vi "LoadStaticConfig.vi"(7 "UIMsg":refnum<class "SendMessage.lvclass">, 8 "error in (no error)":errorcluster, 11 "VXMMotionManager in":refnum<class "VXMMotionManager.lvclass">) -> (0 "error out":errorcluster, 3 "VXMMotionManager out":refnum<class "VXMMotionManager.lvclass">)   [LabVIEW 2018, in "VXMMotionManager.lvclass"]
uses:
  VXMMotionManager.lvclass
  SendMessage/SendMessage.lvclass
  MotionTypes.ctl
  VXMMotionManager.lvclass/VXMMotionManager.ctl
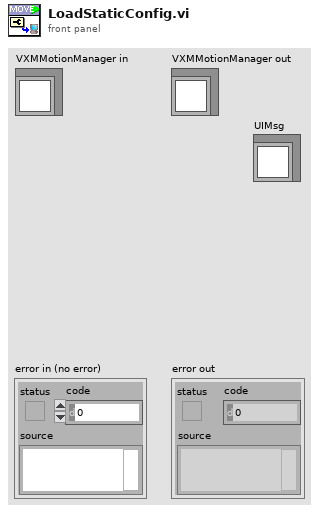
[diagram p1: front panel]
types:
  T1 = typedef "MotionTypes.ctl" = enum16{"Homing", "AllAbsolute", "AllHome", "Position", "OneAxisHome", "Clear"}
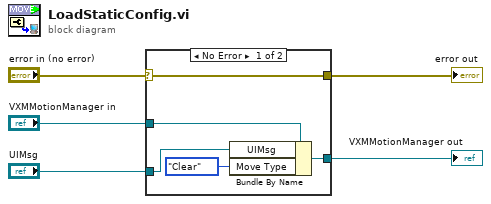
[diagram p0: block diagram]
diagram:
  n1 = case shown="No Error" "error in (no error)" {
    selector: "error in (no error)" -> [w9 w12]
    tunnel: [w9 w12] -> w4
    tunnel: [w8 w11] -> w2
    tunnel: "VXMMotionManager in" -> [w10 w11]
    tunnel: "UIMsg" -> [w7 _]
    frame No Error {
      n2 = Bundle By Name(cluster=w10, "UIMsg"=w7, "Move Type"=MotionTypes."Clear") -> (w8:refnum<class "VXMMotionManager.lvclass">)
    }
    frame Error {
    }
  }
  "error out" <- w4
  "VXMMotionManager out" <- w2
